vi "Read Mesurement Name.vi"(8 "error in (no error)":errorcluster, 11 "Results in":refnum<class "Results.lvclass">) -> (0 "error out":errorcluster, 2 "Measurement":string, 3 "Results out":refnum<class "Results.lvclass">)   [LabVIEW 2015, in "TestStand API.lvlib"]
uses:
  TestStand API.lvlib
  <userlib>/Common Components/Results/Results.lvclass
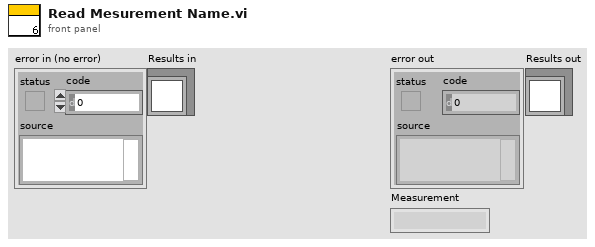
[diagram p1: front panel]
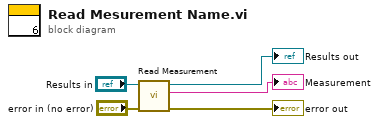
[diagram p0: block diagram]
diagram:
  n1 = call <userlib>:"Read Measurement.vi"("error in (no error)"="error in (no error)", "Results in"="Results in") -> ("error out"=→"error out":errorcluster, "Measurement"=→"Measurement":string, "Results out"=→"Results out":refnum<class "Results.lvclass">)  [unwired: 7 in]
